vi "Configure Waveform Modulation State.vi"(7 "Enable Modulated Output (T: Enable)":bool=TRUE, 8 "error in (no error)":errorcluster, 10 "Waveform Generator Number (1: Waveform Generator 1)":i32(ring)=1 items=["Waveform Generator 1"=1], 11 "VISA resource name":refnum<visa-resource-name>) -> (0 "error out":errorcluster, 3 "VISA resource name out":refnum<visa-resource-name>)   [LabVIEW 2015, in "Agilent 2000 3000 X-Series.lvlib"]
doc: "Enables or disables modulated waveform generator output. You can enable modulation for all waveform generator function types except pulse, DC, and noise."
uses:
  <instrlib>/Agilent 2000 3000 X-Series/Agilent 2000 3000 X-Series.lvlib
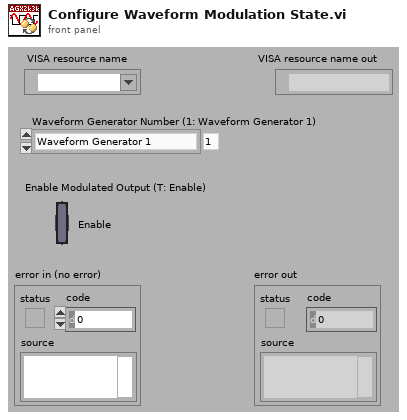
[diagram p1: front panel]
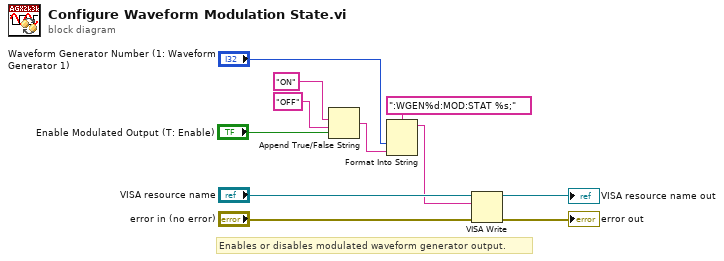
[diagram p0: block diagram]
diagram:
  # "Enables or disables modulated waveform generator output."
  n1 = Append True/False String(1:"Enable Modulated Output (T: Enable)", 2:"OFF", 3:"ON") -> (0:w4:string)  [unwired: 1 out]
  n2 = Format Into String(format string=":WGEN%d:MOD:STAT %s;", "Waveform Generator Number (1: Waveform Generator 1)", w4) -> (resulting string=w1:string)  [unwired: 2 in, 1 out]
  n3 = VISA Write(VISA resource name="VISA resource name", write buffer=w1, error in (no error)="error in (no error)") -> (VISA resource name out=→"VISA resource name out":refnum<visa-resource-name>, error out=→"error out":errorcluster)  [unwired: 1 out]
